vi "002_DataGraph.vi"(11 "Queue Ref In":T1={"UI"=refnum, "Message"=refnum, "Data"=refnum, "Caller"=refnum, "Name"="000 Common", "Data Path"=path "", "Class Path"=path "", "SubPanel"=refnum, "Project Name"="", "MNT"="", "Title"="", "Data Source"=refnum, "Queue List"={}, "VI"=refnum, "UE"=refnum}) -> ()   [LabVIEW 2020]
doc: "000001"
uses:
  Alin/QMH/000 Module Data Type.ctl
  Alin/QMH/Queue Message.ctl
panel:
  in  "Graph":dbl caption="图表时长" format="%#_g s"
  in  "Edit":bool
  in  "Data Graph Edit":bool
  in  "LR":bool
  in  "Start":timestamp caption="开始时间" format="%<%x %.3X>T"
  in  "下拉列表":u16(ring) items=["All"]
  in  "Stop":timestamp caption="结束时间" format="%<%x %.3X>T"
  in  "Operate":i32(listbox) caption="操作日志"
  in  "路径":path
  out "XY图":cluster{"X":dbl, "Y":dbl}[](graph)
  in  "滑动杆":dbl(slide) scale=0.0..10.0
  out "TimeLine":picture
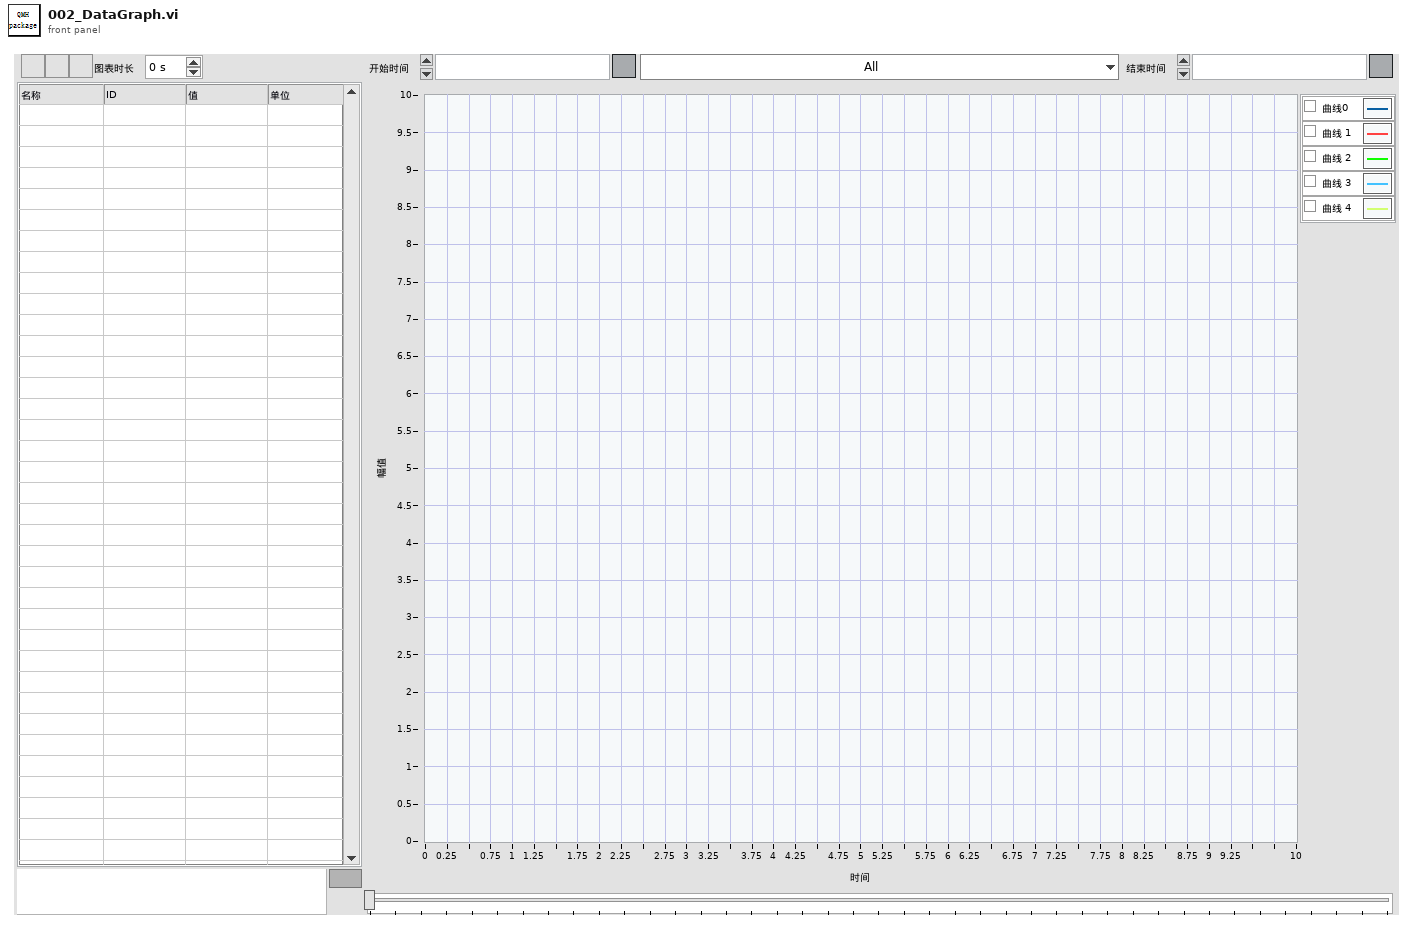
[diagram p1: front panel]
types:
  T1 = typedef "000 Module Data Type.ctl" = cluster{"UI":refnum<queue>, "Message":refnum<queue>, "Data":refnum<queue>, "Caller":refnum<queue>, "Name":string, "Data Path":path, "Class Path":path, "SubPanel":refnum<vi>, "Project Name":string, "MNT":string, "Title":string, "Data Source":refnum<queue>, "Queue List":map{string, refnum<queue>}, "VI":refnum<vi>, "UE":refnum<user-event>}
  T2 = cluster{"Queue":T1, "Delay":cluster{"Count Time(ms)":u32, "Delay Time(ms)":u32, "Next":string}, "Start":refnum<vi>, "Stop":refnum<vi>}
  T3 = typedef "eventvkey.ctl" = enum16{"ASCII", "Enter", "Return", "Shift", "Ctrl", "Alt", "Cmd", "Opt", "Caps", "NumLock", "Clear", "Break", "Up", "Down", "Left", "Right", "Insert", "Delete", "Home", "End", "PageUp", "PageDown", "Escape", "Help", "Pause", "ScrollLock", "F1", "F2", "F3", "F4", "F5", "F6", "F7", "F8", "F9", "F10", "F11", "F12", "F13", "F14", "F15", "F16", "F17", "F18", "F19", "F20", "F21", "F22", "F23", "F24", "Play", "VolumeUp", "VolumeDown", "Mute", "Two Byte Char"}
  T4 = cluster{"Shift":bool, "Ctrl":bool, "Alt":bool, "Cmd":bool, "Opt":bool}
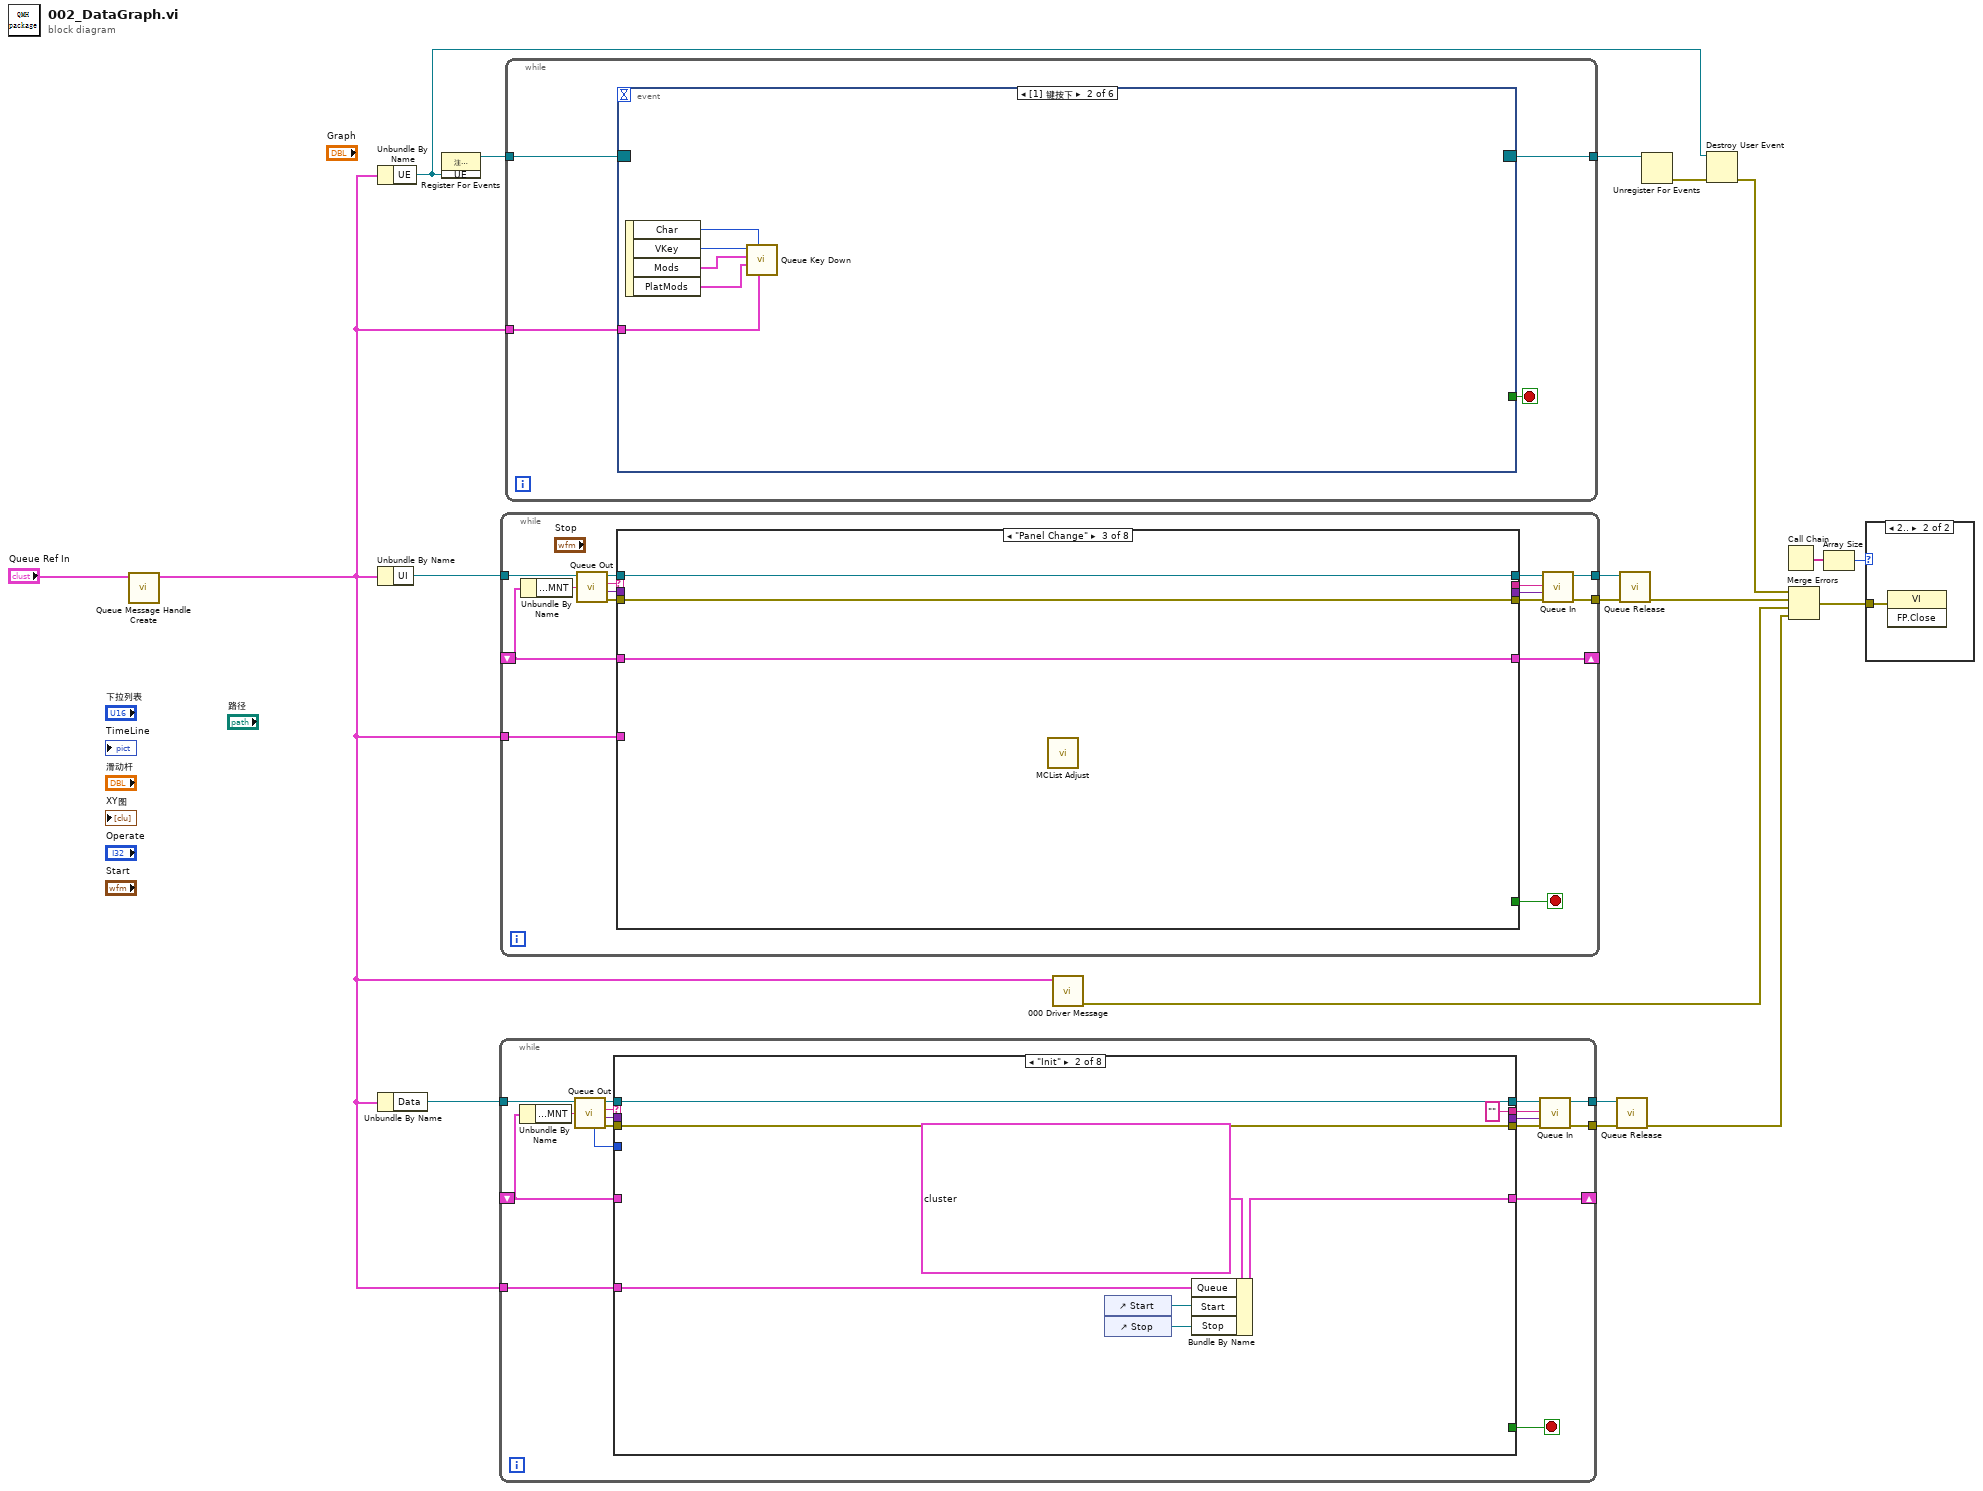
[diagram p0: block diagram]
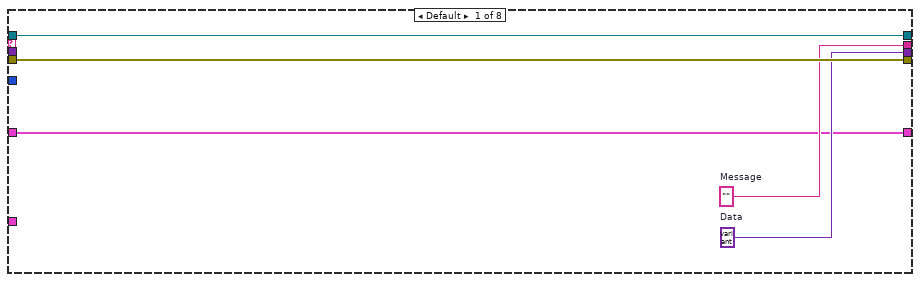
[diagram p2: hidden frame]
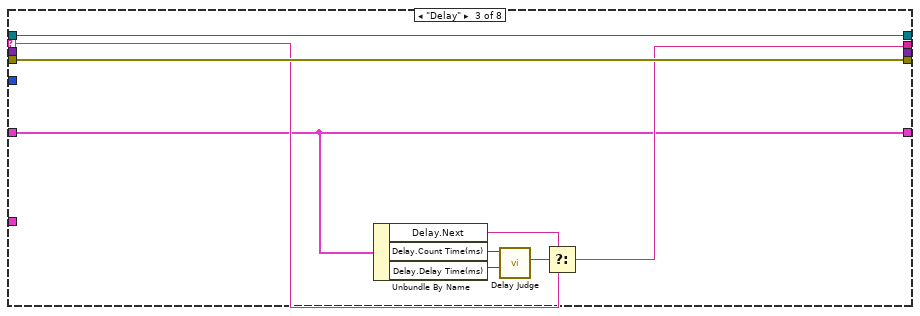
[diagram p3: hidden frame]
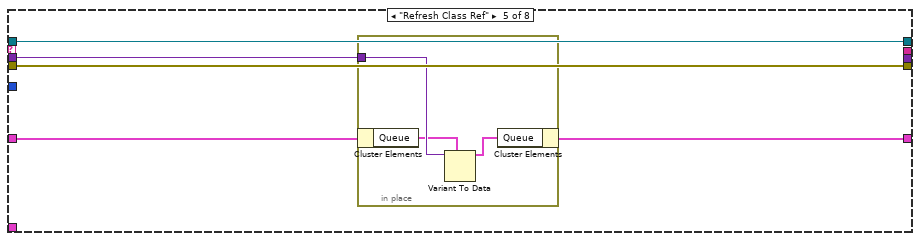
[diagram p5: hidden frame]
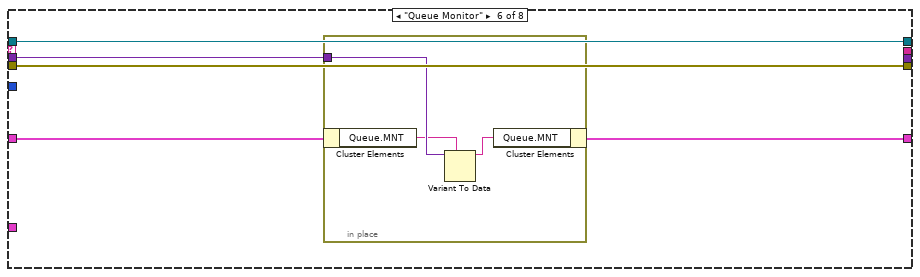
[diagram p6: hidden frame]
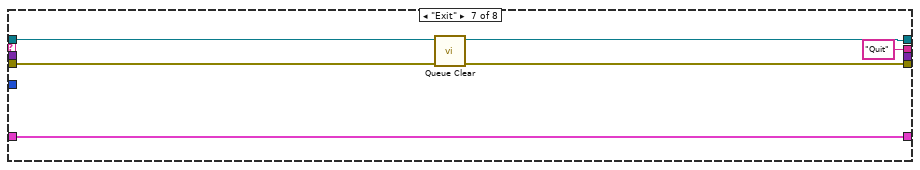
[diagram p7: hidden frame]
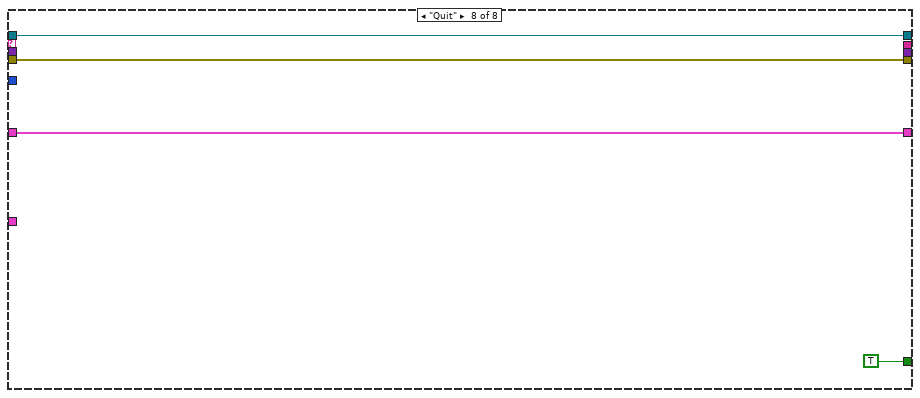
[diagram p8: hidden frame]
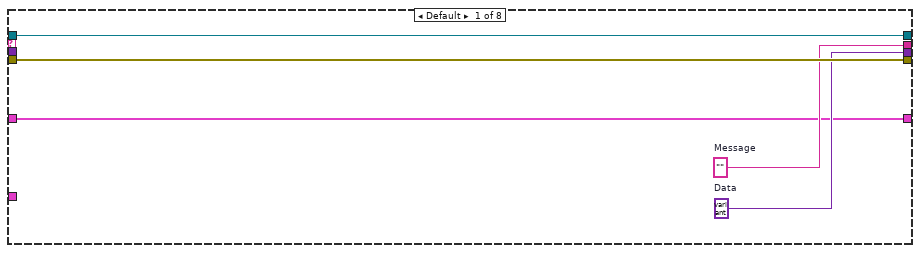
[diagram p10: hidden frame]
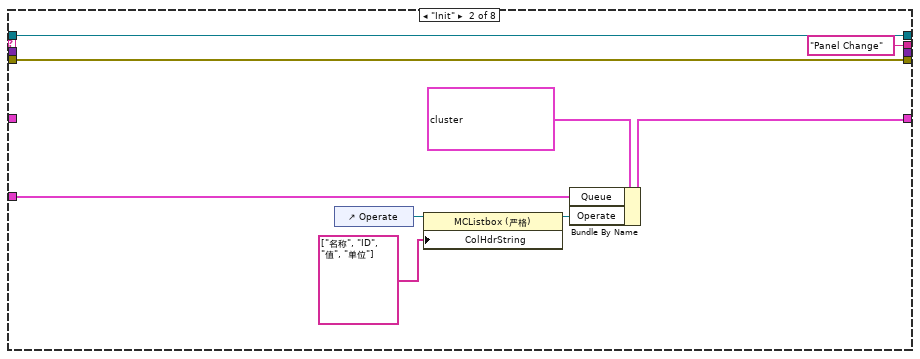
[diagram p11: hidden frame]
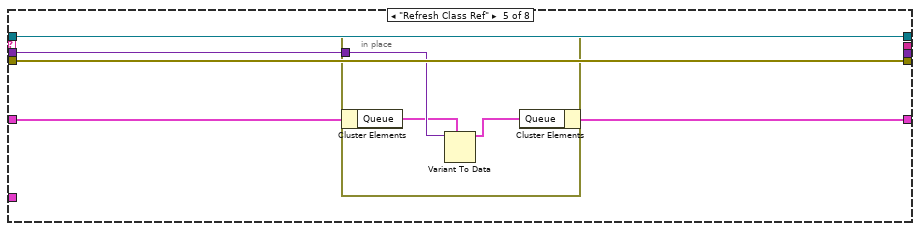
[diagram p13: hidden frame]
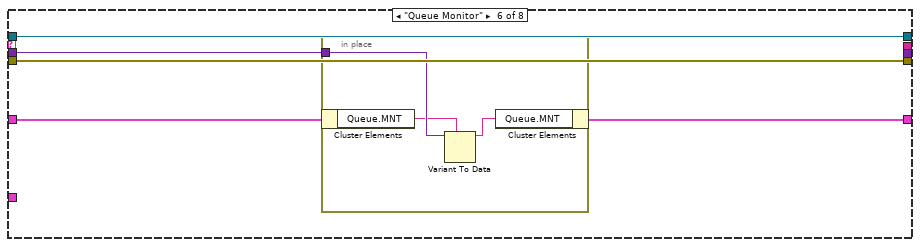
[diagram p14: hidden frame]
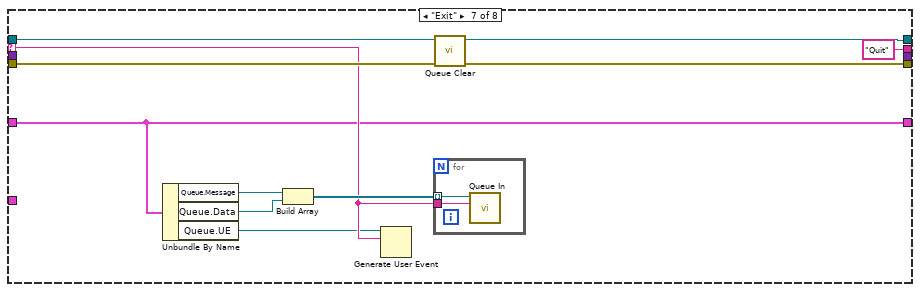
[diagram p15: hidden frame]
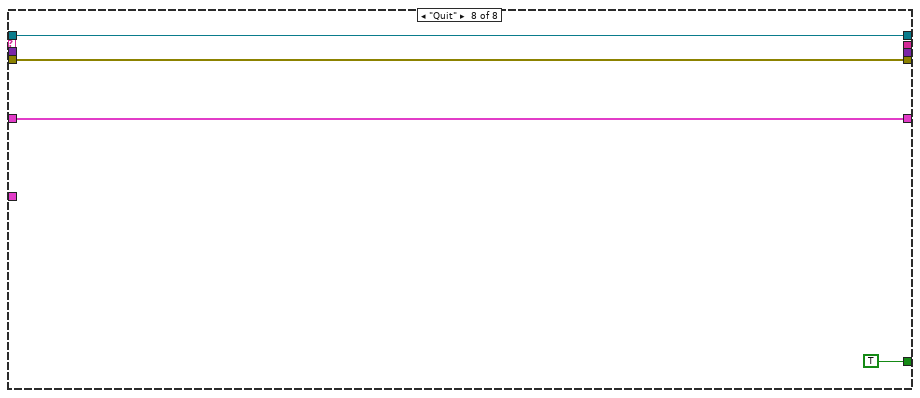
[diagram p16: hidden frame]
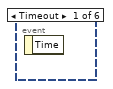
[diagram p17: hidden frame]
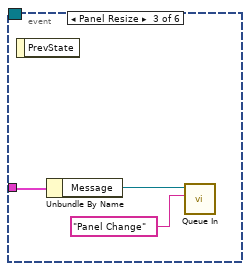
[diagram p18: hidden frame]
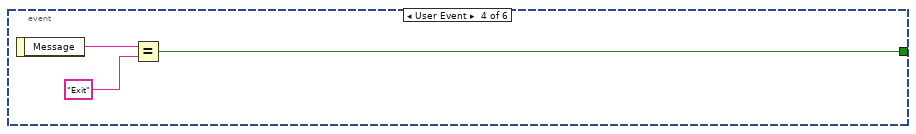
[diagram p19: hidden frame]
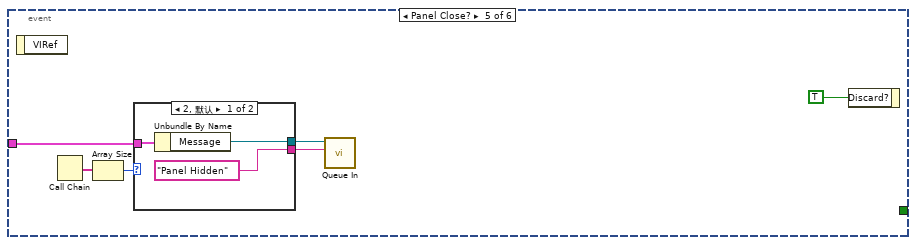
[diagram p20: hidden frame]
diagram:
  n1 = call "Queue Message Handle Create.vi"("Queue Ref In"="Queue Ref In") -> ("Queue Ref Out"=w1:T1)  [unwired: 9 in, 1 out]
  n2 = Unbundle By Name(w1) -> ("UE"=w3:refnum<user-event>)
  n3 = Unbundle By Name(w1) -> ("UI"=w14:refnum<queue>)
  n4 = Unbundle By Name(w1) -> ("Data"=w6:refnum<queue>)
  n5 = register-events(w3) -> (reference out=w19:refnum<event-registration>)  [unwired: 2 in, 1 out]
  n6 = while {
    tunnel: w6 -> [w32]
    tunnel: [w29] -> w8
    tunnel: [w28] -> w7
    shift-right: [w24] -> _
    shift-left: _ -> [w21]
    tunnel: w1 -> [w20]
    stop <- w36 stop-if-true
    n7 = Unbundle By Name(w21) -> ("Queue.MNT"=w22:string)
    n8 = call "Queue Out.vi"("Monitor"=w22, "Queue In"=w32) -> ("error out"=w35:errorcluster, "Data"=w33:variant, "Message"=w34:string, "Queue Out"=w31:refnum<queue>, "Queue NUmber"=w23:i32)  [unwired: 5 in]
    n9 = case shown="\"Init\"" w34 {
      selector: w34 -> [_ _ w51 _ _ _ _ _]
      tunnel: w31 -> [w41 w49 w58 w61 w66 w74 w82 w86]
      tunnel: w35 -> [w40 w48 w57 w60 w65 w73 w80 w87]
      tunnel: [w41 w49 w58 w61 w66 w74 w81 w86] -> w30
      tunnel: [w40 w48 w57 w60 w65 w73 w79 w87] -> w27
      tunnel: [w39 "" ("Next") w52 _ _ _ "Quit" _] -> w26
      tunnel: [_ _ _ _ _ _ _ TRUE] -> w36
      tunnel: [w38 _ _ _ _ _ _ _] -> w25
      tunnel: w33 -> [_ _ _ _ w62 w70 _ _]
      tunnel: [w37 w45 w50 w59 w63 w71 w78 w84] -> w24
      tunnel: w21 -> [w37 _ w50 w59 w64 w72 w78 w84]
      tunnel: w23 -> [_ _ _ _ _ _ _ _]
      tunnel: w20 -> [_ w44 _ _ _ _ _ _]
      frame Default {
        w38 = variant  # Data
        w39 = ""  # Message
      }
      frame "Init" {
        n10 = control-ref of="Start"() -> (w43:refnum<vi>)
        n11 = control-ref of="Stop"() -> (w42:refnum<vi>)
        n12 = Bundle By Name(cluster=T2 {"Queue"={"UI"=refnum, "Message"=refnum, "Data"=refnum, "Caller"=refnum, "Name"="000 Common", "Data Path"=path "", "Class Path"=path "", "SubPanel"=refnum, "Project Name"="", "MNT"="", "Title"="", "Data Source"=refnum, "Queue List"={}, "VI"=refnum, "UE"=refnum}, "Delay"={"Count Time(ms)"=250, "Delay Time(ms)"=250, "Next"="Receive Data,Delay"}, "Start"=refnum, "Stop"=refnum}, "Queue"=w44, "Start"=w43, "Stop"=w42) -> (w45:T2)
      }
      frame "Delay" {
        n13 = Unbundle By Name(w50) -> ("Delay.Next"=w56:string, "Delay.Count Time(ms)"=w53:u32, "Delay.Delay Time(ms)"=w54:u32)
        n14 = call "Delay Judge.vi"("Delay Time(ms)"=w54, "Count Time(ms)"=w53) -> ("Time Out?"=w55:bool)  [unwired: 5 in, 4 out]
        n15 = Select(t=w56, s=w55, f=w51) -> (s? t:f=w52:string)
      }
      frame "====System====" {
      }
      frame "Refresh Class Ref" {
        n16 = in-place {
          in-place-border: w62 -> [w69]
          n17 = in-place-cluster #1(w64) -> ("Queue"=w68:T1)
          n18 = Variant To Data(type=w68, Variant=w69) -> (data=w67:T1)  [unwired: 1 in, 1 out]
          n19 = in-place-cluster #1("Queue"=w67) -> (w63:T2)
        }
      }
      frame "Queue Monitor" {
        n20 = in-place {
          in-place-border: w70 -> [w77]
          n21 = in-place-cluster #2(w72) -> ("Queue.MNT"=w76:string)
          n22 = Variant To Data(type=w76, Variant=w77) -> (data=w75:string)  [unwired: 1 in, 1 out]
          n23 = in-place-cluster #2("Queue.MNT"=w75) -> (w71:T2)
        }
      }
      frame "Exit" {
        n24 = call "Queue Clear.vi"("error in (no error)"=w80, "Queue In"=w82) -> ("error out"=w79:errorcluster, "Queue Out"=w81:refnum<queue>)  [unwired: 8 in]
      }
      frame "Quit" {
      }
    }
    n25 = call "Queue In.vi"("error in (no error)"=w27, "Data"=w25, "Message"=w26, "Queue In"=w30) -> ("error out"=w28:errorcluster, "Queue Out"=w29:refnum<queue>)  [unwired: 6 in]
  }
  n26 = while {
    tunnel: w14 -> [w99]
    tunnel: [w96] -> w16
    tunnel: [w95] -> w15
    shift-right: [w91] -> _
    shift-left: _ -> [w90]
    tunnel: w1 -> [w88]
    stop <- w103 stop-if-true
    n27 = Unbundle By Name(w90) -> ("Queue.MNT"=w89:string)
    n28 = call "Queue Out.vi"("Monitor"=w89, "Queue In"=w99) -> ("error out"=w102:errorcluster, "Data"=w100:variant, "Message"=w101:string, "Queue Out"=w98:refnum<queue>)  [unwired: 5 in, 1 out]
    n29 = case shown="\"Panel Change\"" w101 {
      selector: w101 -> [_ _ _ _ _ _ w142 _]
      tunnel: w98 -> [w108 w117 w120 w123 w128 w136 w149 w155]
      tunnel: w102 -> [w107 w116 w119 w122 w127 w135 w147 w156]
      tunnel: [w108 w117 w120 w123 w128 w136 w148 w155] -> w97
      tunnel: [w107 w116 w119 w122 w127 w135 w146 w156] -> w94
      tunnel: [w106 "Panel Change" ("Message") _ _ _ _ "Quit" _] -> w93
      tunnel: [_ _ _ _ _ _ _ TRUE] -> w103
      tunnel: [w105 _ _ _ _ _ _ _] -> w92
      tunnel: w100 -> [_ _ _ _ w124 w132 _ _]
      tunnel: [w104 w114 w118 w121 w125 w133 w141 w153] -> w91
      tunnel: w90 -> [w104 _ w118 w121 w126 w134 w141 w153]
      tunnel: w88 -> [_ w113 _ _ _ _ _ _]
      frame Default {
        w105 = variant  # Data
        w106 = ""  # Message
      }
      frame "Init" {
        n30 = control-ref of="Operate"() -> (w112:refnum<vi>)
        n31 = property class="MCListbox (严格)"(reference=w112, "ColHdrString"=string[] ["名称", "ID", "值", "单位"] ("列首字符串[]")) -> (reference out=w111:refnum<vi>)  [unwired: 1 in, 1 out]
        n32 = Bundle By Name(cluster=cluster{"Queue":T1, "Operate":refnum<vi>} {"Queue"={"UI"=refnum, "Message"=refnum, "Data"=refnum, "Caller"=refnum, "Name"="000 Common", "Data Path"=path "", "Class Path"=path "", "SubPanel"=refnum, "Project Name"="", "MNT"="", "Title"="", "Data Source"=refnum, "Queue List"={}, "VI"=refnum, "UE"=refnum}, "Operate"=refnum}, "Queue"=w113, "Operate"=w111) -> (w114:cluster{"Queue":T1, "Operate":refnum<vi>})
      }
      frame "Panel Change" {
        n33 = call "MCList Adjust.vi"() -> ()  [unwired: 11 in, 1 out]
      }
      frame "====System====" {
      }
      frame "Refresh Class Ref" {
        n34 = in-place {
          in-place-border: w124 -> [w131]
          n35 = in-place-cluster #3(w126) -> ("Queue"=w130:T1)
          n36 = Variant To Data(type=w130, Variant=w131) -> (data=w129:T1)  [unwired: 1 in, 1 out]
          n37 = in-place-cluster #3("Queue"=w129) -> (w125:cluster{"Queue":T1, "Operate":refnum<vi>})
        }
      }
      frame "Queue Monitor" {
        n38 = in-place {
          in-place-border: w132 -> [w139]
          n39 = in-place-cluster #4(w134) -> ("Queue.MNT"=w138:string)
          n40 = Variant To Data(type=w138, Variant=w139) -> (data=w137:string)  [unwired: 1 in, 1 out]
          n41 = in-place-cluster #4("Queue.MNT"=w137) -> (w133:cluster{"Queue":T1, "Operate":refnum<vi>})
        }
      }
      frame "Exit" {
        n42 = Unbundle By Name(w141) -> ("Queue.Message"=w145:refnum<queue>, "Queue.Data"=w144:refnum<queue>, "Queue.UE"=w140:refnum<user-event>)
        n43 = Build Array(w145, w144) -> (w143:refnum<queue>[])
        n44 = Generate User Event(user event=w140, event data cluster=w142) -> ()  [unwired: 2 in, 2 out]
        n45 = for {
          tunnel: w143 -> [w152] mode=indexing
          tunnel: w142 -> [w151]
          n46 = call "Queue In.vi"("Message"=w151, "Queue In"=w152) -> ()  [unwired: 8 in, 2 out]
        }
        n47 = call "Queue Clear.vi"("error in (no error)"=w147, "Queue In"=w149) -> ("error out"=w146:errorcluster, "Queue Out"=w148:refnum<queue>)  [unwired: 8 in]
      }
      frame "Quit" {
      }
    }
    n48 = call "Queue In.vi"("error in (no error)"=w94, "Data"=w92, "Message"=w93, "Queue In"=w97) -> ("error out"=w95:errorcluster, "Queue Out"=w96:refnum<queue>)  [unwired: 6 in]
  }
  n49 = while {
    tunnel: w19 -> [w160]
    tunnel: [w158] -> w18
    tunnel: w1 -> [w157]
    stop <- w159 stop-if-true
    n50 = event shown="[1] 键按下" {
      selector: w160 -> [_ _ _ _ _ _]
      dyn-events: [_ _ _ _ _ _] -> w158
      timeout: _ -> [_ _ _ _ _ _]
      tunnel: [_ _ _ w169 _ _] -> w159
      tunnel: w157 -> [_ w164 w168 _ w174 _]
      event Timeout {
        n51 = event-data() -> ()  [unwired: 1 in, 1 out]
      }
      event Key Down {
        n52 = event-data() -> ("Char"=w165:i16, "VKey"=w163:T3, "Mods"=w162:cluster{"Num Pad":bool, "Menu Key":bool}, "PlatMods"=w161:T4)  [unwired: 1 in]
        n53 = call "Queue Key Down.vi"("Queue Ref Out"=w164, "C"=w165, "Platform Key"=w161, "Group Key"=w162, "V Key"=w163) -> ()  [unwired: 6 in, 1 out]
      }
      event Panel Resize {
        n54 = event-data() -> ()  [unwired: 1 in, 1 out]
        n55 = Unbundle By Name(w168) -> ("Message"=w167:refnum<queue>)
        n56 = call "Queue In.vi"("Message"="Panel Change", "Queue In"=w167) -> ()  [unwired: 8 in, 2 out]
      }
      event User Event {
        n57 = event-data() -> ("Message"=w171:string)  [unwired: 1 in]
        n58 = Equal?(x=w171, y="Exit") -> (x = y?=w169:bool)
      }
      event Panel Close? {
        n59 = event-data() -> ()  [unwired: 1 in, 1 out]
        n60 = Call Chain() -> (call chain=w176:string[])
        n61 = Array Size(array=w176) -> (size(s)=w175:i32)
        n62 = case shown="2, 默认" w175 {
          tunnel: w174 -> [w180 w183]
          tunnel: [w179 w182] -> w173
          tunnel: ["Panel Hidden" ("Message") "Exit Prepare" ("Message")] -> w172
          frame 2, Default {
            n63 = Unbundle By Name(w180) -> ("Message"=w179:refnum<queue>)
          }
          frame 1 {
            n64 = Unbundle By Name(w183) -> ("Message"=w182:refnum<queue>)
          }
        }
        n65 = call "Queue In.vi"("Message"=w172, "Queue In"=w173) -> ()  [unwired: 8 in, 2 out]
        n66 = event-data("Discard?"=TRUE ("放弃？")) -> ()  [unwired: 1 in, 1 out]
      }
      event "Data Graph Edit", "LR", "Edit": Value Change {
        n67 = event-data() -> ("CtlRef"=w184:refnum<vi>)  [unwired: 1 in]
        n68 = property class="Bool" props=["Label", "Text"](reference=w184) -> ()  [unwired: 1 in, 3 out]
      }
    }
  }
  n69 = call "000 Driver Message.vi"("Queue In"=w1) -> ("error out"=w4:errorcluster)  [unwired: 8 in, 2 out]
  n70 = call "Queue Release.vi"("error in (no error)"=w7, "Queue In"=w8) -> ("error out"=w5:errorcluster)  [unwired: 9 in]
  n71 = call "Queue Release.vi"("error in (no error)"=w15, "Queue In"=w16) -> ("error out"=w12:errorcluster)  [unwired: 9 in]
  n72 = Unregister For Events(event registration refnum=w18) -> (error out=w17:errorcluster)  [unwired: 1 in]
  n73 = Destroy User Event(user event=w3, error in=w17) -> (error out=w13:errorcluster)
  n74 = Call Chain() -> (call chain=w10:string[])
  n75 = Merge Errors(w13, w12, w4, w5) -> (w11:errorcluster)
  n76 = Array Size(array=w10) -> (size(s)=w9:i32)
  n77 = case shown="2.." w9 {
    tunnel: w11 -> [_ w185]
    frame 0, Default {
    }
    frame 2.. {
      n78 = invoke class="VI" method="FP.Close"(error in=w185) -> ()  [unwired: 2 in, 3 out]
    }
  }
